vi "SetPortArmAngle.vi"(8 "error in (no error)":errorcluster, 10 "Ticks":dbl) -> (0 "error out":errorcluster)   [LabVIEW 2015]
uses:
  Framework/Motor Ref Names Type Def.ctl
  <vilib>/Rock Robotics/WPI/CAN/TalonSRX/WPI_CANTalonSRX_APIControlMode.ctl
  Framework/Robot Global Data.vi
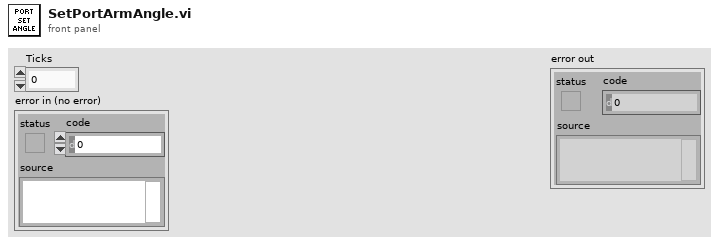
[diagram p1: front panel]
types:
  T1 = typedef "WPI_CANTalonSRX_APIControlMode.ctl" = enum8{"Percent VBus", "Speed", "Position", "Slave", "Unchanged / Invalid", "Voltage Compensation", "Current", "Motion Profile"}
  T2 = typedef "Motor Ref Names Type Def.ctl" = enum16{"Angular Motor", "Shooter Motor Bottom", "Shooter Motor Top", "Arm Shooter Motor"}
  T3 = typedef "Motor Ref Array Type Def.ctl" = T4[]
  T4 = typedef "Detailed Motor Type Def.ctl" = cluster{"MotorRef":T5, "Encoder Ticks Per Rev":dbl, "Set Position":dbl}
  T5 = typedef "WPI_MotorControlDeviceRef.ctl" = cluster{"DeviceStatus":errorcluster, "Type":T6, "PWM":cluster{"PWM Channel":T7, "DeadBand":T8}, "CAN":cluster{"Device Number":u8, "Control Mode":T9, "Semaphore":T10, "Max Vout":dbl, "TalonSRX Control Mode":T1}, "Invert":bool}
  T6 = typedef "WPI_MotorControlType.ctl" = enum16{"PWM", "CAN", "CANTalonSRX"}
  T7 = typedef "FPGA_DIOPWMChannel.ctl" = enum8{"PWM 0", "PWM 1", "PWM 2", "PWM 3", "PWM 4", "PWM 5", "PWM 6", "PWM 7", "PWM 8", "PWM 9", "PWM MXP 0", "PWM MXP 1", "PWM MXP 2", "PWM MXP 3", "PWM MXP 4", "PWM MXP 5", "PWM MXP 6", "PWM MXP 7", "PWM MXP 8", "PWM MXP 9", "Invalid"}
  T8 = typedef "WPI_PWMDeadband.ctl" = cluster{"Name":string, "maxPositivePwm":i32, "minPositivePwm":i32, "centerPwm":i32, "maxNegativePwm":i32, "minNegativePwm":i32, "angularRange":u16}
  T9 = typedef "WPI_CANJaguar_ControlMode.ctl" = enum8{"Percent VBus", "Current", "Speed", "Position", "Voltage"}
  T10 = typedef "Semaphore RefNum" = refnum<k1>
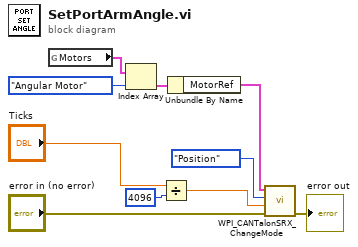
[diagram p0: block diagram]
diagram:
  n1 = global read "Robot Global Data.vi" "Motors"() -> (w10:T3)
  n2 = Index Array(array=w10, index=Motor_Ref_Names_Type_Def."Angular Motor" ("Motor Ref Names")) -> (element=w8:T4)
  n3 = Divide(x="Ticks", y=4096) -> (x/y=w4:dbl)
  n4 = Unbundle By Name(w8) -> ("MotorRef"=w5:T5)
  n5 = call <vilib>:"WPI_CANTalonSRX_ChangeMode.vi"("error in (no error)"="error in (no error)", "Output"=w4, "Control Mode"=WPI_CANTalonSRX_APIControlMode."Position", "CAN Talon SRX Ref"=w5) -> ("error out"=→"error out":errorcluster)  [unwired: 6 in, 1 out]
